vi "CSM - Convert Argument to Error.vi"(4 "Argument":string) -> (1 "Error":errorcluster)   [LabVIEW 2017, in "Communicable State Machine.lvlib"]
doc: "Converts the CSM error argument format to a LabVIEW Error Cluster.\n\n\n> [!NOTE] <b>CSM Argument Type</b>\n>\n> In CSM, all arguments and return values are presented in string format, but they can carry any data type underneath. Therefore, the sender must encode first, and the receiver must decode afterwards. For example, CSM has a built-in HEXSTR encoding scheme, and custom codecs can also be extended as needed. To facilitate the identification of the encoding method, it is recommended to write the encoded argument in the format `<Argument Type> STRING FORMAT ARGUMENT`. Use the CSM - Argument Type VI to extract the type tag and select the corresponding decoding function accordingly.\n\n\n> [!NOTE] <b>CSM ERRSTR Format Argument</b>\n>\n> The LabVIEW Error Cluster is a complex data type. The error information string usually contains carriage returns, which cannot be directly passed as a CSM argument. Although error cluster information can be converted to HEXSTR format, this method lacks readability, making it impossible to read information intuitively in logs. Therefore, to pass LabVIEW error information in CSM arguments, CSM has a built-in ERRSTR format argument encoding/decoding scheme. The argument type string is ERRSTR. The conversion process is as follows:\n>\n> 1. Format the code and source in the error cluster into a string with the following format:\n>\n> Error: `<ERRSTR>[Error: error-code] error-description-As-safe-argument-string`\n> Warning: `<ERRSTR>[Warning: error-code] warning-description-As-safe-argument-string`\n>\n> 2. Replace special characters in this string with safe characters.\n>\n> 3. Obtain the CSM ERRSTR format argument, which can be safely embedded in the state string without disrupting CSM message parsing.\n\n\n<b>Reference Example</b>: `[CSM-Example]\\0. Base Concepts\\4.2 Arguments - Error As Arguments.vi`.\n\n-- <b>Controls</b> --\n- <b>Argument</b>: CSM error argument format.\n\n-- <b>Indicators</b> --\n- <b>Error</b>: LabVIEW Error Cluster."
uses:
  Communicable State Machine.lvlib
  CSM - Keywords.vi
  _Shared/CSM Shared.lvlib
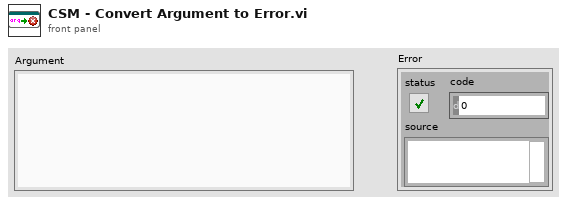
[diagram p1: front panel]
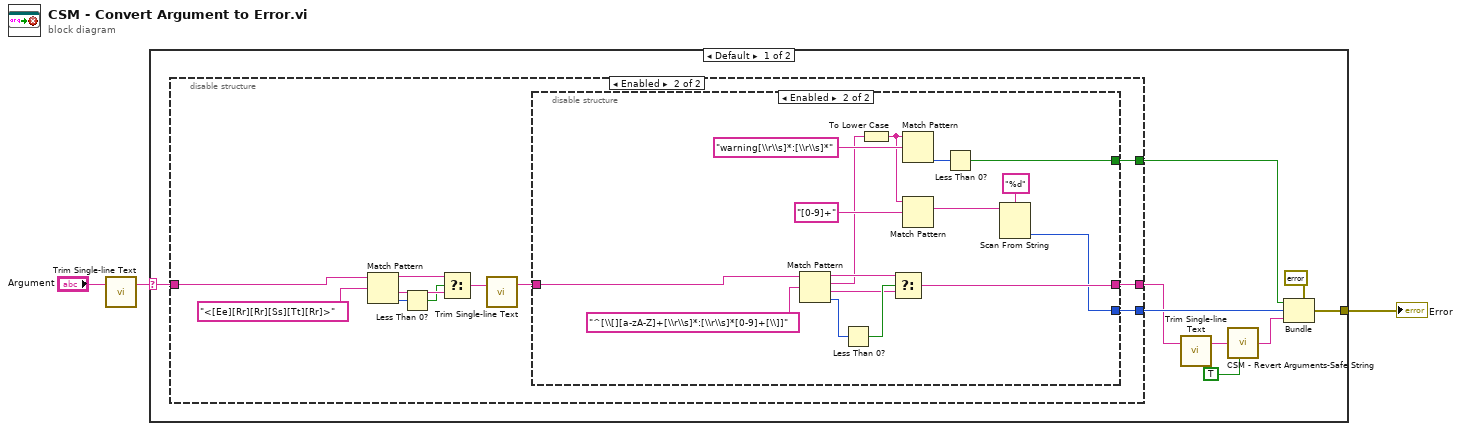
[diagram p0: block diagram]
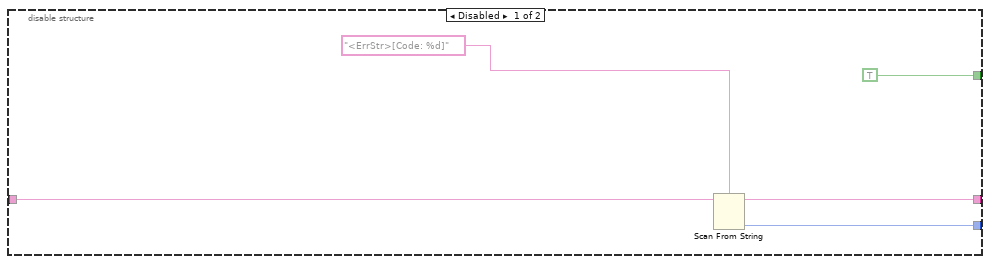
[diagram p2: hidden frame]
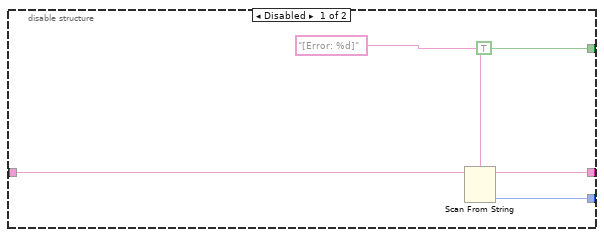
[diagram p3: hidden frame]
diagram:
  n1 = call "Trim Single-line Text.vi"("single-line text"="Argument") -> ("trimed text"=w2:string)  [unwired: 2 in]
  n2 = case shown="Default" w2 {
    selector: w2 -> [w6 _]
    tunnel: [w10 _] -> w1
    frame Default {
      n3 = disable-structure shown="Enabled" {
        disable-tunnel: [w16 w25] -> w11
        disable-tunnel: [w15 w26] -> w8
        disable-tunnel: w6 -> [w14 w27]
        disable-tunnel: [TRUE ("status") w18] -> w5
        frame Disabled {
          n4 = Scan From String(format string="<ErrStr>[Code: %d]", input string=w14) -> (remaining string=w15:string, output 1=w16:i32)  [unwired: 3 in, 2 out]
        }
        frame Enabled {
          n5 = Match Pattern(string=w27, regular expression="<[Ee][Rr][Rr][Ss][Tt][Rr]>") -> (before substring=w22:string, after substring=w23:string, offset past match=w24:i32)  [unwired: 1 in, 1 out]
          n6 = Less Than 0?(x=w24) -> (x < 0?=w21:bool)
          n7 = Select(t=w22, s=w21, f=w23) -> (s? t:f=w20:string)
          n8 = call "Trim Single-line Text.vi"("single-line text"=w20) -> ("trimed text"=w19:string)  [unwired: 2 in]
          n9 = disable-structure shown="Enabled" {
            disable-tunnel: [w32 w43] -> w26
            disable-tunnel: [w31 w38] -> w25
            disable-tunnel: w19 -> [w30 w49]
            disable-tunnel: [TRUE ("status") w40] -> w18
            frame Disabled {
              n10 = Scan From String(format string="[Error: %d]", input string=w30) -> (remaining string=w32:string, output 1=w31:i32)  [unwired: 3 in, 2 out]
            }
            frame Enabled {
              n11 = Match Pattern(string=w49, regular expression="^[\\[][a-zA-Z]+[\\r\\s]*:[\\r\\s]*[0-9]+[\\]]") -> (before substring=w44:string, match substring=w36:string, after substring=w45:string, offset past match=w46:i32)  [unwired: 1 in]
              n12 = Less Than 0?(x=w46) -> (x < 0?=w47:bool)
              n13 = To Lower Case(string=w36) -> (all lower case string=w35:string)
              n14 = Select(t=w44, s=w47, f=w45) -> (s? t:f=w43:string)
              n15 = Match Pattern(string=w35, regular expression="warning[\\r\\s]*:[\\r\\s]*") -> (offset past match=w41:i32)  [unwired: 1 in, 3 out]
              n16 = Match Pattern(string=w35, regular expression="[0-9]+") -> (match substring=w34:string)  [unwired: 1 in, 3 out]
              n17 = Less Than 0?(x=w41) -> (x < 0?=w40:bool)
              n18 = Scan From String(format string="%d", input string=w34) -> (output 1=w38:i32)  [unwired: 3 in, 3 out]
            }
          }
        }
      }
      n19 = call "Trim Single-line Text.vi"("single-line text"=w8) -> ("trimed text"=w7:string)  [unwired: 2 in]
      n20 = call "CSM - Revert Arguments-Safe String.vi"("Safe Argument String"=w7, "Force Convert (F)"=TRUE) -> ("Origin Argument String"=w9:string)  [unwired: 7 in]
      n21 = Bundle(cluster=errorcluster {"status"=TRUE, "code"=0, "source"=""} ("error in (no error)"), "status"=w5, "code"=w11, "source"=w9) -> (w10:errorcluster)
    }
    frame "" {
    }
  }
  "Error" <- w1
